vi "UTIL Launch Asynchronous Process.vi"(8 "error in (no error)":errorcluster, 9 "Timeout (5s)":dbl=5.0, 10 "Arguments":string, 11 "Process Path":path) -> (0 "error out":errorcluster, 3 "Standard Output":string)   [LabVIEW 2015, in "niDTS CommLib.lvlib" / "niDTS Comm EXE.lvclass"]
doc: "Launches a process (executable, application) at the specified <b>Process Path</b>, taking care to pass in any <b>Arguments</b>, and then kills the process if a specified <b>Timeout</b> is reached."
uses:
  niDTS Comm EXE.lvclass
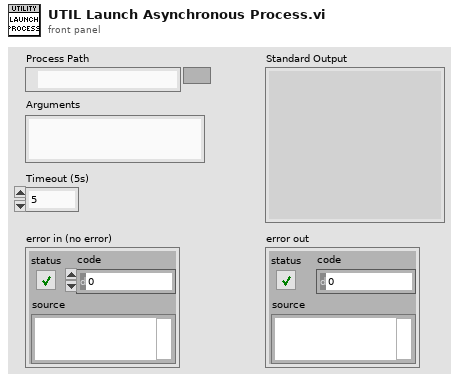
[diagram p1: front panel]
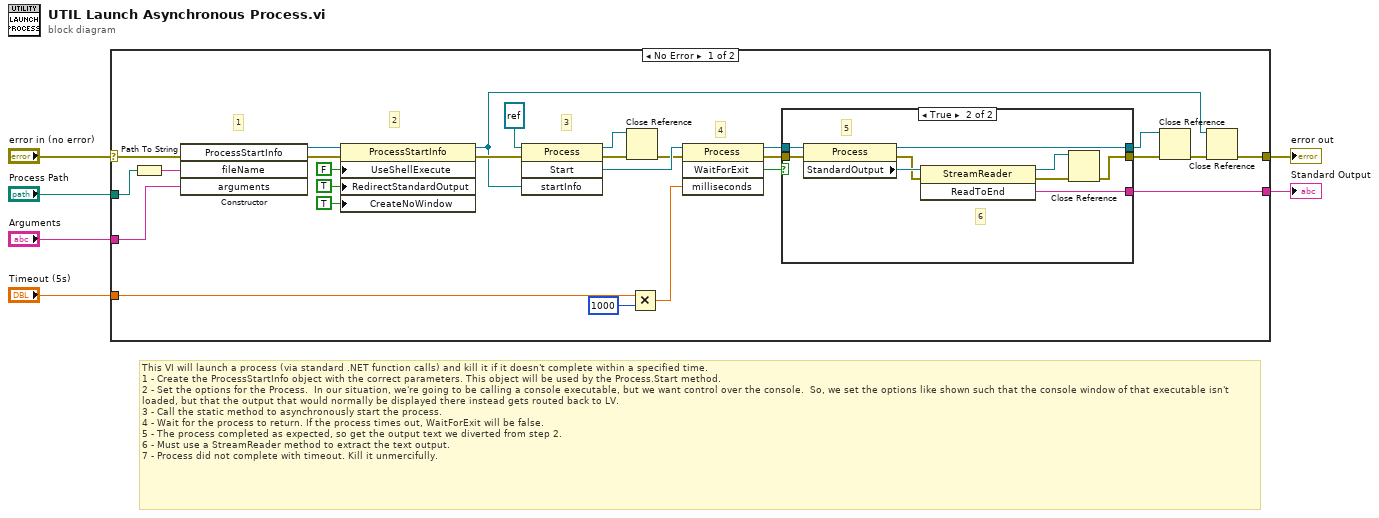
[diagram p0: block diagram]
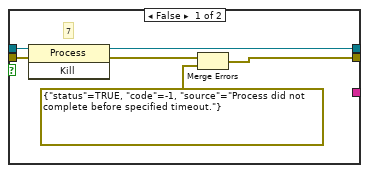
[diagram p2: hidden frame]
diagram:
  # "This VI will launch a process (via standard .NET function calls) and kill it if it doesn't complete within a specified time.\n1 - Create the ProcessStartInfo object with the correct parameters. This object will be used by the Process.Start method. \n2 - Set the options for the Process.  In our situation, we're going to be calling a console executable, but we want control over the console.  So, we set the options like shown such that the console window of that executable isn't loaded, but that the output that would normally be displayed there instead gets routed back to LV.\n3 - Call the static method to asynchronously start the process.\n4 - Wait for the process to return. If the process times out, WaitForExit will be false.\n5 - The process completed as expected, so get the output text we diverted from step 2.\n6 - Must use a StreamReader method to extract the text output.\n7 - Process did not complete with timeout. Kill it unmercifully."
  n1 = case shown="No Error" "error in (no error)" {
    selector: "error in (no error)" -> [w19 w49]
    tunnel: "Process Path" -> [w30 _]
    tunnel: "Arguments" -> [w20 _]
    tunnel: [w9 w49] -> w4
    tunnel: "Timeout (5s)" -> [w28 _]
    tunnel: [w8 _] -> w1
    frame No Error {
      # "4"
      # "3"
      # "2"
      # "1"
      n2 = Path To String(path=w30) -> (string=w21:string)
      n3 = constructor class="ProcessStartInfo"(error in=w19, "fileName"=w21, "arguments"=w20) -> (reference out=w16:refnum<k24>, error out=w18:errorcluster)  [unwired: 2 in, 3 out]
      n4 = property class="ProcessStartInfo"(reference=w16, error in=w18, "UseShellExecute"=FALSE, "RedirectStandardOutput"=TRUE, "CreateNoWindow"=TRUE) -> (reference out=w10:refnum<k24>, error out=w17:errorcluster)
      n5 = invoke class="Process" method="Start"(reference=refnum<k24> refnum ("new reference"), error in=w17, "startInfo"=w10) -> (reference out=w33:refnum<k24>, error out=w32:errorcluster, "Start"=w29:refnum<k24>)  [unwired: 1 in, 1 out]
      n6 = Close Reference(reference=w33, error in (no error)=w32) -> (error out=w25:errorcluster)
      n7 = Multiply(x=w28, y=1000) -> (x*y=w26:dbl)
      n8 = invoke class="Process" method="WaitForExit"(reference=w29, error in=w25, "milliseconds"=w26) -> (reference out=w24:refnum<k24>, error out=w23:errorcluster, "WaitForExit"=w22:bool)  [unwired: 1 in, 1 out]
      n9 = case shown="True" w22 {
        tunnel: w24 -> [w39 w43]
        tunnel: w23 -> [w38 w44]
        tunnel: [w35 w42] -> w12
        tunnel: [w34 w41] -> w11
        tunnel: [_ w40] -> w8
        frame False {
          # "7"
          n10 = invoke class="Process" method="Kill"(reference=w39, error in=w38) -> (reference out=w35:refnum<k24>, error out=w37:errorcluster)  [unwired: 1 in, 1 out]
          n11 = Merge Errors(w37, errorcluster {"status"=TRUE, "code"=-1, "source"="Process did not complete before specified timeout."} ("error out")) -> (w34:errorcluster)
        }
        frame True {
          # "6"
          # "5"
          n12 = property class="Process"(reference=w43, error in=w44) -> (reference out=w42:refnum<k24>, error out=w47:errorcluster, "StandardOutput"=w48:refnum<k24>)
          n13 = invoke class="StreamReader" method="ReadToEnd"(reference=w48, error in=w47) -> (reference out=w46:refnum<k24>, error out=w45:errorcluster, "ReadToEnd"=w40:string)  [unwired: 1 in]
          n14 = Close Reference(reference=w46, error in (no error)=w45) -> (error out=w41:errorcluster)
        }
      }
      n15 = Close Reference(reference=w12, error in (no error)=w11) -> (error out=w13:errorcluster)
      n16 = Close Reference(reference=w10, error in (no error)=w13) -> (error out=w9:errorcluster)
    }
    frame Error {
    }
  }
  "error out" <- w4
  "Standard Output" <- w1
